vi "Queue_Create.vi"   [LabVIEW 2020]
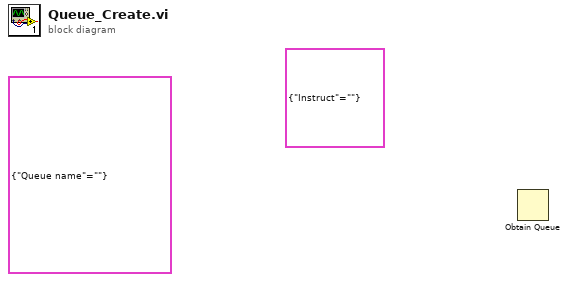
[diagram p0: block diagram]
diagram:
  (unwired) cluster{"Instruct":string} {"Instruct"=""}
  (unwired) cluster{"Queue name":string} {"Queue name"=""}
  n1 = Obtain Queue() -> ()  [unwired: 5 in, 3 out]
